vi "Configure Multi Eval Meas Limit EVM.vi"(4 "Peak (60.0)":dbl=60.0 format="%^.3e", 5 "Peak Enabled (Off)":i32(ring) items=["Off", "On", "Value"], 6 "RMS (30.0)":dbl=30.0 format="%^.3e", 7 "RMS Enabled (Off)":i32(ring) items=["Off", "On", "Value"], 8 "error in (no error)":errorcluster, 9 "Modulation (Pi/2-BPSK)":i32(ring) items=["Pi/2-BPSK", "QPSK", "16-QAM", "64-QAM", "256-QAM"], 10 "Instance (1)":T1=1, 11 "VISA resource name":refnum<visa-resource-name>) -> (0 "error out":errorcluster, 3 "VISA resource name out":refnum<visa-resource-name>)   [LabVIEW 2015, in "Rohde&Schwarz CMXP NR FR2 Measurement.lvlib"]
doc: "Defines upper limits for the RMS and peak values of the error vector magnitude (EVM) for selected modulation scheme.\n\nAttributes:\nRSCMXPNRFR2M_ATTR_MULTI_EVAL_MEASUREMENT_LIMIT_PHBPSK_EVM\nRSCMXPNRFR2M_ATTR_MULTI_EVAL_MEASUREMENT_LIMIT_QPSK_EVM\nRSCMXPNRFR2M_ATTR_MULTI_EVAL_MEASUREMENT_LIMIT_QAM16_EVM\nRSCMXPNRFR2M_ATTR_MULTI_EVAL_MEASUREMENT_LIMIT_QAM64_EVM\nRSCMXPNRFR2M_ATTR_MULTI_EVAL_MEASUREMENT_LIMIT_QAM256_EVM\n\nRemote-control commands:\nCONFigure:NRMMw:MEAS<i>:MEValuation:LIMit:PHBPsk:EVMagnitude\nCONFigure:NRMMw:MEAS<i>:MEValuation:LIMit:QPSK:EVMagnitude\nCONFigure:NRMMw:MEAS<i>:MEValuation:LIMit:QAM<order>:EVMagnitude"
uses:
  <instrlib>/Rohde&Schwarz CMXP NR FR2 Measurement/Rohde&Schwarz CMXP NR FR2 Measurement.lvlib
  <instrlib>/Rohde&Schwarz CMXP NR FR2 Measurement/Private/_Instance.ctl
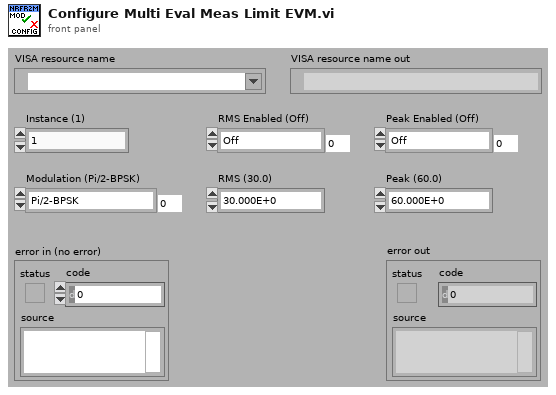
[diagram p1: front panel]
types:
  T1 = typedef "Rohde&Schwarz CMXP NR FR2 Measurement.lvlib/_Instance.ctl" = i32
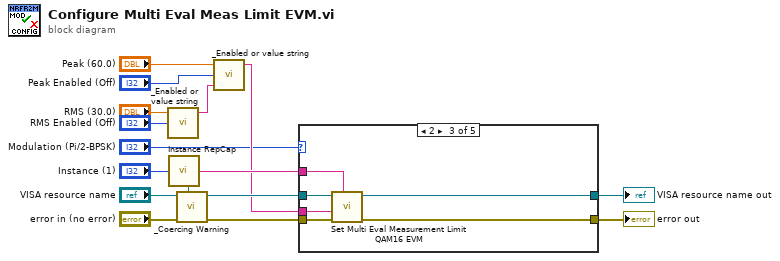
[diagram p0: block diagram]
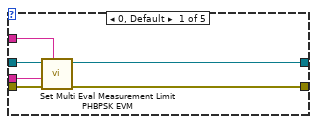
[diagram p2: hidden frame]
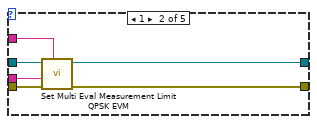
[diagram p3: hidden frame]
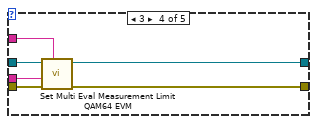
[diagram p4: hidden frame]
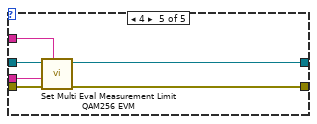
[diagram p5: hidden frame]
diagram:
  n1 = call <instrlib>:"_Enabled or value string.vi"("Enabled or Value"="RMS Enabled (Off)", "Value"="RMS (30.0)") -> ("Resulting String"=w3:string)  [unwired: 3 in]
  n2 = call <instrlib>:"Instance RepCap.vi"("Instance In"="Instance (1)") -> ("In Range?"=w13:bool, "RepCap Identifier Out"=w9:string)  [unwired: 1 in]
  n3 = call <instrlib>:"_Coercing Warning.vi"("In Range?"=w13, "error in (no error)"="error in (no error)", "VISA resource name"="VISA resource name") -> ("error out"=w10:errorcluster, "VISA resource name out"=w11:refnum<visa-resource-name>)  [unwired: 7 in]
  n4 = call <instrlib>:"_Enabled or value string.vi"("Initial String"=w3, "Enabled or Value"="Peak Enabled (Off)", "Value"="Peak (60.0)") -> ("Resulting String"=w8:string)  [unwired: 2 in]
  n5 = case shown="2" "Modulation (Pi/2-BPSK)" {
    tunnel: w11 -> [w22 w28 w34 w40 w46]
    tunnel: w10 -> [w21 w27 w33 w39 w45]
    tunnel: w9 -> [w20 w26 w32 w38 w44]
    tunnel: w8 -> [w17 w23 w29 w35 w41]
    tunnel: [w19 w25 w31 w37 w43] -> w7
    tunnel: [w18 w24 w30 w36 w42] -> w6
    frame 0, Default {
      n6 = call "Set Multi Eval Measurement Limit PHBPSK EVM"("Repeated Capabilities"=w20, "error in (no error)"=w21, "Multi Eval Measurement Limit PHBPSK EVM ()"=w17, "instrument handle"=w22) -> ("error out"=w19:errorcluster, "instrument handle out"=w18:refnum<visa-resource-name>)  [unwired: 6 in]
    }
    frame 1 {
      n7 = call "Set Multi Eval Measurement Limit QPSK EVM"("Repeated Capabilities"=w26, "error in (no error)"=w27, "Multi Eval Measurement Limit QPSK EVM ()"=w23, "instrument handle"=w28) -> ("error out"=w25:errorcluster, "instrument handle out"=w24:refnum<visa-resource-name>)  [unwired: 6 in]
    }
    frame 2 {
      n8 = call "Set Multi Eval Measurement Limit QAM16 EVM"("Repeated Capabilities"=w32, "error in (no error)"=w33, "Multi Eval Measurement Limit QAM16 EVM ()"=w29, "instrument handle"=w34) -> ("error out"=w31:errorcluster, "instrument handle out"=w30:refnum<visa-resource-name>)  [unwired: 6 in]
    }
    frame 3 {
      n9 = call "Set Multi Eval Measurement Limit QAM64 EVM"("Repeated Capabilities"=w38, "error in (no error)"=w39, "Multi Eval Measurement Limit QAM64 EVM ()"=w35, "instrument handle"=w40) -> ("error out"=w37:errorcluster, "instrument handle out"=w36:refnum<visa-resource-name>)  [unwired: 6 in]
    }
    frame 4 {
      n10 = call "Set Multi Eval Measurement Limit QAM256 EVM"("Repeated Capabilities"=w44, "error in (no error)"=w45, "Multi Eval Measurement Limit QAM256 EVM ()"=w41, "instrument handle"=w46) -> ("error out"=w43:errorcluster, "instrument handle out"=w42:refnum<visa-resource-name>)  [unwired: 6 in]
    }
  }
  "error out" <- w7
  "VISA resource name out" <- w6
